vi "lisa_functional_5.vi"   [LabVIEW 2019]
doc: "The classic \"Hello World\" example."
uses:
  <vilib>/Analysis/Matrix/Datatypes/ComplexMatrix.ctl
  <vilib>/Platform/TimedLoop/XDataNode/timing_clust.ctl
  <vilib>/Platform/TimedLoop/XDataNode/nitl_modes.ctl
  <vilib>/Platform/TimedLoop/XDataNode/wakeup.ctl
  <vilib>/platform/TimedLoop/XDataNode/XDataNode.xnode
  <vilib>/Platform/TimedLoop/XDataNode/XDNodeRunTimeDep.lvlib
  <vilib>/Analysis/Matrix/NI_Matrix.lvlib
types:
  T1 = typedef "imagedata.ctl" = cluster{"image type":i32, "image depth":i32, "image":u8[], "mask":u8[], "colors":u32[], "Rectangle":cluster{"left":i16, "top":i16, "right":i16, "bottom":i16}}
  T2 = typedef "XDNodeRunTimeDep.lvlib/timing_clust.ctl" = cluster{"Expected End [f-1]":u64, "Actual End [f-1]":u64, "Finished Late? [f-1]":bool, "Expected End [i-1]":u64, "Actual End [i-1]":u64, "Finished Late? [i-1]":bool, "Expected Start [i]":u64, "Actual Start [i]":u64, "Expected Start [f]":u64, "Actual Start [f]":u64, "Source Name":string, "Structure Name":string, "Period":i64, "Deadline":i64, "Offset":i64, "Start":i64, "Priority":i32, "Timeout":i32, "Mode":T3, "Wakeup Reason":T4, "Error":errorcluster, "Source Type":string, "Secondary Source Type":string, "Global End Time":u64, "Global Start Time":u64, "Frame Duration":u64, "Iteration Duration":u64, "Assigned CPU":i32, "I/O Scan Engine Mode":u32}
  T3 = typedef "XDNodeRunTimeDep.lvlib/nitl_modes.ctl" = enum32{"No Change", "Process missed periods, maintain original phase", "Discard missed periods, maintain original phase", "Process missed periods, ignore original phase", "Discard missed periods, ignore original phase"}
  T4 = typedef "XDNodeRunTimeDep.lvlib/wakeup.ctl" = enum32{"Normal", "Aborted", "Asynchronous wakeup", "Timing source error", "Timed loop error", "Timeout"}
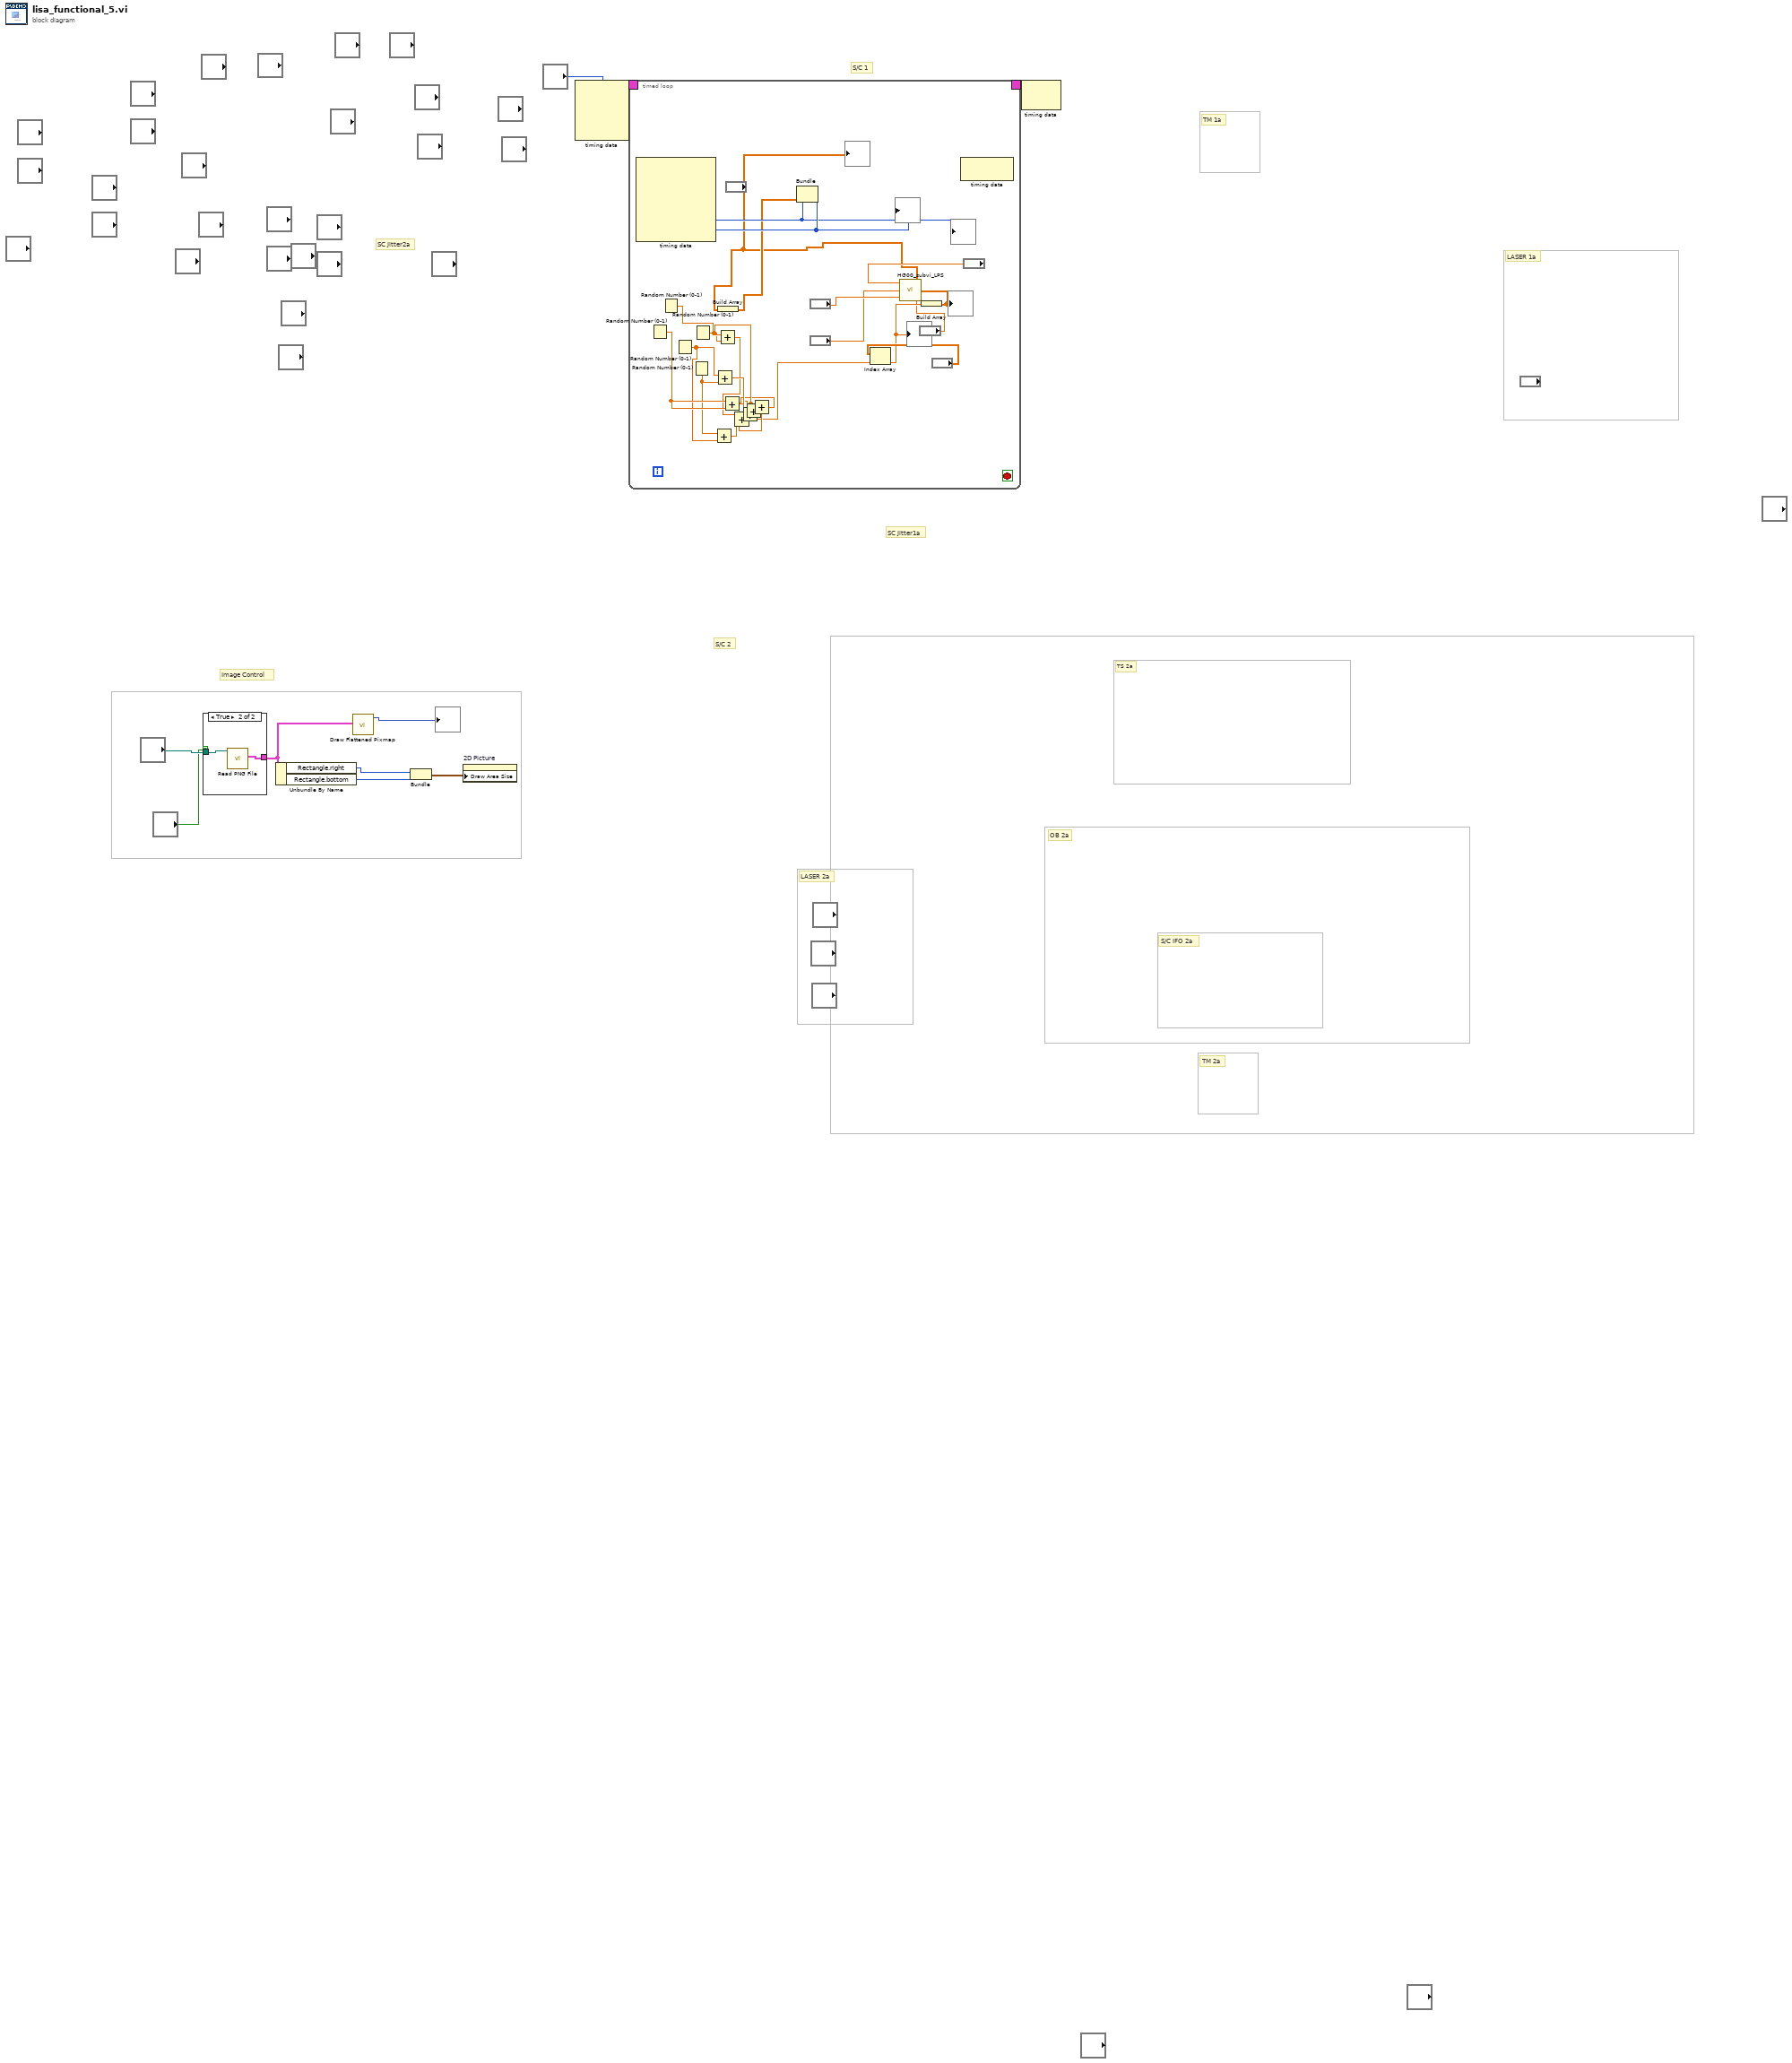
[diagram p0: block diagram]
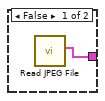
[diagram p2: hidden frame]
diagram:
  # "SC Jitter1a"
  # "SC Jitter2a"
  # "S/C IFO 2a"
  # "TM 2a"
  # "TS 2a"
  # "OB 2a"
  # "S/C 2"
  # "TM 1a"
  # "LASER 2a"
  # "Image Control"
  # "LASER 1a"
  # "S/C 1"
  n1 = case shown="True" "?" {
    tunnel: "?" -> [_ w13]
    tunnel: [w11 w12] -> w7
    frame False {
      n2 = call <vilib>:"Read JPEG File.vi"() -> ("image data"=w11:T1)  [unwired: 9 in, 2 out]
    }
    frame True {
      n3 = call <vilib>:"Read PNG File.vi"("path to PNG file"=w13) -> ("image data"=w12:T1)  [unwired: 8 in, 2 out]
    }
  }
  n4 = Unbundle By Name(w7) -> ("Rectangle.right"=w9:i16, "Rectangle.bottom"=w8:i16)
  n5 = call <vilib>:"Draw Flattened Pixmap.vi"("image data"=w7) -> ("new picture"=→"?":picture)  [unwired: 8 in]
  n6 = Bundle("right"=w9, "bottom"=w8) -> (w5:cluster{"right":i16, "bottom":i16})  [unwired: 1 in]
  n7 = property on="2D Picture" class="Pict"("Draw Area Size"=w5) -> ()  [unwired: 2 in, 2 out]
  n8 = node-c288("?") -> (w3:T2)  [unwired: 3 in]
  n9 = timed-loop {
    timing: w3 -> [_]
    timing-out: [_] -> w2
    stop <- _ stop-if-true
    n10 = node-c288() -> (w28:i64, w29:i64)  [unwired: 1 in, 5 out]
    "?" <- w29
    "?" <- w28
    n11 = Random Number (0-1)() -> (number: 0 to 1=w24:dbl)
    n12 = Random Number (0-1)() -> (number: 0 to 1=w25:dbl)
    n13 = Random Number (0-1)() -> (number: 0 to 1=w22:dbl)
    n14 = Random Number (0-1)() -> (number: 0 to 1=w23:dbl)
    n15 = Random Number (0-1)() -> (number: 0 to 1=w21:dbl)
    n16 = Add(x=w23, y=w22) -> (x+y=w17:dbl)
    n17 = Add(x=w22, y=w23) -> (x+y=w20:dbl)
    n18 = Add(x=w25, y=w21) -> (x+y=w19:dbl)
    n19 = Add(x=w24, y=w24) -> (x+y=w18:dbl)
    n20 = Add(x=w18, y=w17) -> (x+y=w15:dbl)
    n21 = Add(x=w20, y=w19) -> ()  [unwired: 1 out]
    n22 = Add(x=w21, y=w21) -> (x+y=w16:dbl)
    n23 = Add(x=w16, y=w15) -> (x+y=w14:dbl)
    n24 = Index Array(array="?", index=w14) -> (element=w35:dbl)
    "?" <- w35
    n25 = Build Array(w35) -> (w34:dbl[])
    "?" <- w34
    n26 = call "HG00_subvi_LPS.vi"("Shift"="?", "Tilt"=w34, "w"="?", "l"="?", "Gap"="?") -> ("return value 2"=w26:dbl[])
    "?" <- w26
    n27 = Build Array(w26) -> (w27:dbl[][])
    n28 = Bundle("Actual Start [i]"=w28, "Period"=w29, w27) -> ()  [unwired: 1 in, 1 out]
    n29 = node-c288() -> ()  [unwired: 1 in, 1 out]
  }
  n30 = node-c288(w2) -> ()  [unwired: 1 out]
